vi "Read Power Instruments.vi"(8 "error in (no error)":errorcluster, 11 "Supervisor in":refnum<class "Supervisor.lvclass">) -> (0 "error out":errorcluster, 2 "Power Instruments":T1={"HPR"=FALSE, "Sonar 1"=TRUE, "Sonar 2"=TRUE, "Doppler"=TRUE, "Laser"=FALSE, "KRAFT"=FALSE, "Pan/Tilt"=FALSE, "Transponder"=FALSE, "Still Cam"=FALSE, "HD Cam"=FALSE, "UHI Cam"=FALSE}, 3 "Supervisor out":refnum<class "Supervisor.lvclass">)   [LabVIEW 2014, in "Supervisor.lvclass"]
uses:
  Supervisor.lvclass
  Supervisor.lvclass/Supervisor.ctl
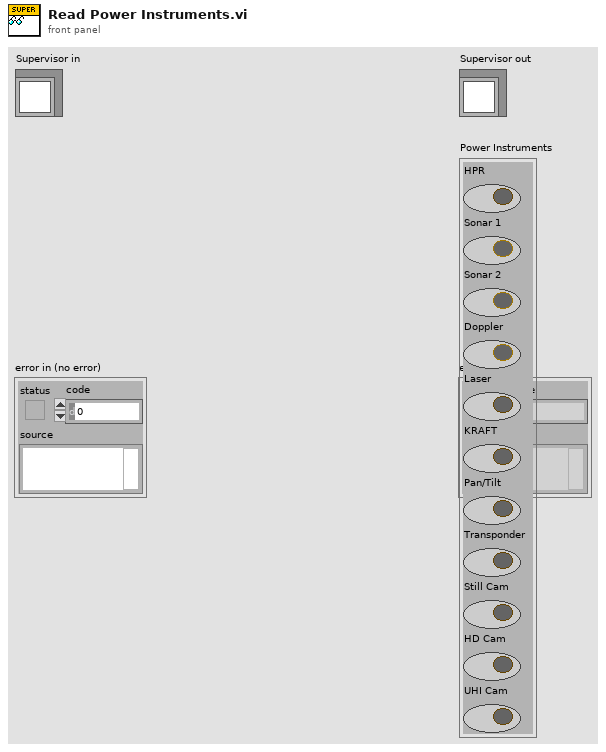
[diagram p1: front panel]
types:
  T1 = cluster{"HPR":bool, "Sonar 1":bool, "Sonar 2":bool, "Doppler":bool, "Laser":bool, "KRAFT":bool, "Pan/Tilt":bool, "Transponder":bool, "Still Cam":bool, "HD Cam":bool, "UHI Cam":bool}
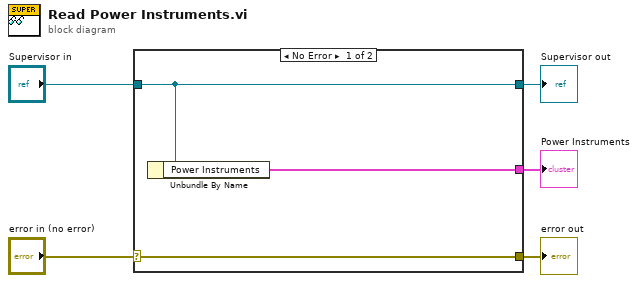
[diagram p0: block diagram]
diagram:
  n1 = case shown="No Error" "error in (no error)" {
    selector: "error in (no error)" -> [w8 w9]
    tunnel: [w8 w9] -> w4
    tunnel: [w7 w10] -> w2
    tunnel: "Supervisor in" -> [w7 w10]
    tunnel: [w6 _] -> w1
    frame No Error {
      n2 = Unbundle By Name(w7) -> ("Power Instruments"=w6:T1)
    }
    frame Error {
    }
  }
  "error out" <- w4
  "Supervisor out" <- w2
  "Power Instruments" <- w1
